vi "LoadRAWdataV2.0.vi"(2 "pos offset (0)":i32, 3 "action":enum16{"OPEN", "READ", "CLOSE", "DATASREENER"}(ring)) -> (0 "RAW data":T1, 1 "error out":errorcluster)   [LabVIEW 2009]
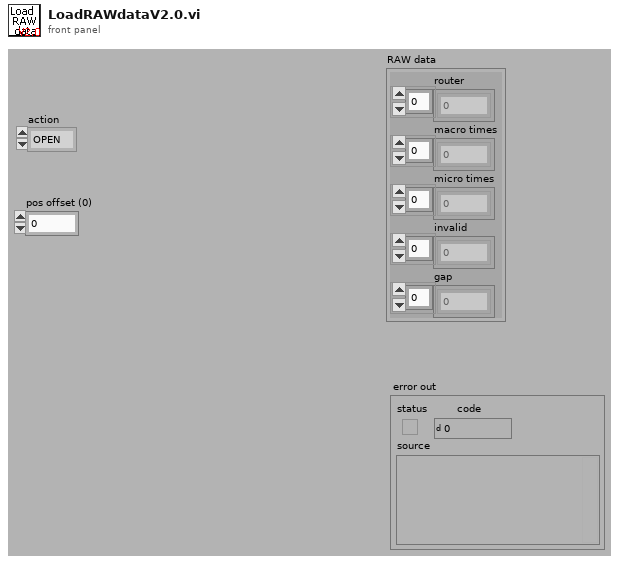
[diagram p1: front panel]
types:
  T1 = cluster{"router":u8[], "macro times":dbl[], "micro times":u16[], "invalid":dbl[], "gap":dbl[]}
  T2 = enum16{"read/write", "read-only", "write-only", "write-only (truncate)"}
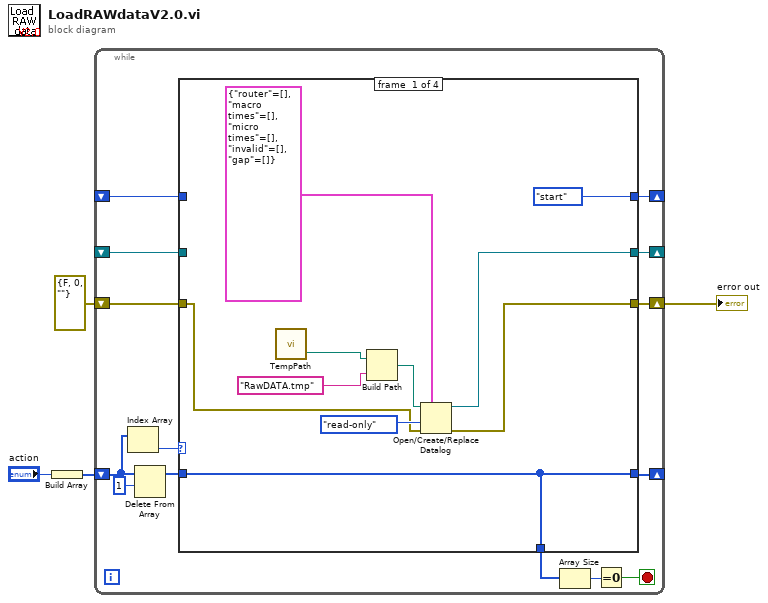
[diagram p0: block diagram]
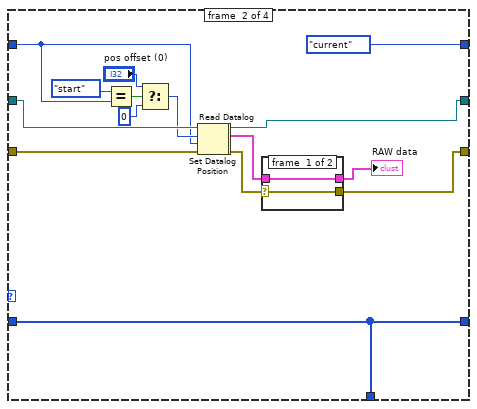
[diagram p2: hidden frame]
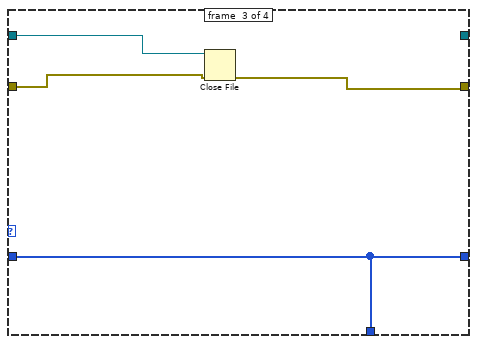
[diagram p4: hidden frame]
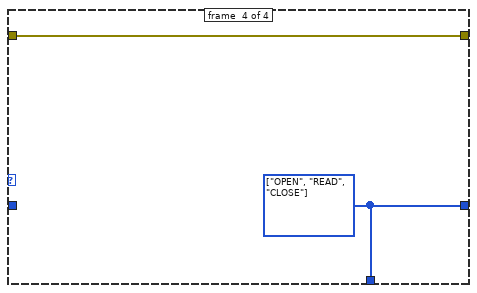
[diagram p5: hidden frame]
diagram:
  n1 = Build Array("action") -> (w1:enum16{"OPEN", "READ", "CLOSE", "DATASREENER"}[])
  n2 = while {
    shift-right: [w18] -> _
    shift-left: _ -> [w16]
    shift-right: [w17] -> w4
    shift-left: errorcluster {"status"=FALSE, "code"=0, "source"=""} ("error out") -> [w15]
    shift-right: [w14] -> _
    shift-left: _ -> [w13]
    shift-right: [w10] -> _
    shift-left: w1 -> [w7]
    stop <- w11 stop-if-true
    n3 = Index Array(array=w7) -> (element=w8:enum16{"OPEN", "READ", "CLOSE", "DATASREENER"})  [unwired: 1 in]
    n4 = Delete From Array(array=w7, length=1) -> (array with subset deleted=w5:enum16{"OPEN", "READ", "CLOSE", "DATASREENER"}[])  [unwired: 1 in, 1 out]
    n5 = case shown="\"OPEN\"" w8 {
      tunnel: [w23 w43 _ _] -> w18
      tunnel: [w22 w34 w51 w55] -> w17
      tunnel: w16 -> [_ w44 w53 _]
      tunnel: w15 -> [w20 w45 w52 w55]
      tunnel: [enum16{"start", "end", "current"}."start" ("pos mode (0:2)") enum16{"start", "end", "current"}."current" ("pos mode (0:2)") _ _] -> w14
      tunnel: w13 -> [_ w36 _ _]
      tunnel: [w19 w31 w50 w54] -> w10
      tunnel: [w19 w31 w50 w54] -> w9
      tunnel: w5 -> [w19 w31 w50 _]
      frame #0 {
        n6 = call "TempPath.vi"() -> ("stripped path 2"=w28:path)  [unwired: 3 in]
        n7 = Build Path(base path=w28, name or relative path="RawDATA.tmp") -> (appended path=w26:path)
        n8 = Open/Create/Replace Datalog(5:T1 {"router"=[], "macro times"=[], "micro times"=[], "invalid"=[], "gap"=[]} ("cluster"), 8:w20, 9:T2."read-only" ("open mode (0)"), 11:w26) -> (0:w22:errorcluster, 3:w23:refnum<k1>)  [unwired: 2 in, 1 out]
      }
      frame #1 {
        n9 = Equal?(x=enum16{"start", "end", "current"}."start", y=w36) -> (x = y?=w40:bool)
        n10 = Select(t="pos offset (0)", s=w40, f=0 ("pos offset (0)")) -> (s? t:f=w37:i32)
        n11 = Set Datalog Position(4:w45, 5:w36, 6:w37, 7:w44) -> (0:w29:errorcluster, 3:w30:refnum<k1>)
        n12 = Read Datalog(4:w29, 7:w30) -> (0:w35:errorcluster, 2:w33:T1, 3:w43:refnum<k1>)  [unwired: 1 in]
        n13 = case shown="No Error" w35 {
          selector: w35 -> [w47 w49]
          tunnel: [w47 w49] -> w34
          tunnel: w33 -> [w46 w48]
          tunnel: [w46 w48] -> w32
          frame #0 {
          }
          frame #1 {
          }
        }
        "RAW data" <- w32
      }
      frame #2 {
        n14 = Close File(refnum=w53, error in=w52) -> (error out=w51:errorcluster)  [unwired: 1 out]
      }
      frame #3 {
        w54 = enum16{"OPEN", "READ", "CLOSE", "DATASREENER"}[] [enum."OPEN", enum."READ", enum."CLOSE"] items=["OPEN", "READ", "CLOSE", "DATASREENER"]
      }
    }
    n15 = Array Size(array=w9) -> (size(s)=w12:i32)
    n16 = Equal To 0?(x=w12) -> (x = 0?=w11:bool)
  }
  "error out" <- w4
